vi "Get All Algorithms Info.vi"(6 "Backend engine":T1, 8 "error in":errorcluster) -> (0 "error out":errorcluster, 3 "All Algorithms Info":T2[](array[typedef]))   [LabVIEW 2013, in "QWTBLVLib.lvlib"]
doc: "Get informations on all available Algorithms."
uses:
  QWTBLVLib.lvlib
  TD Algorithm Information.ctl
  TD Algorithm Information Input.ctl
  TD Algorithm Information Output.ctl
  TD Backend Engine.ctl
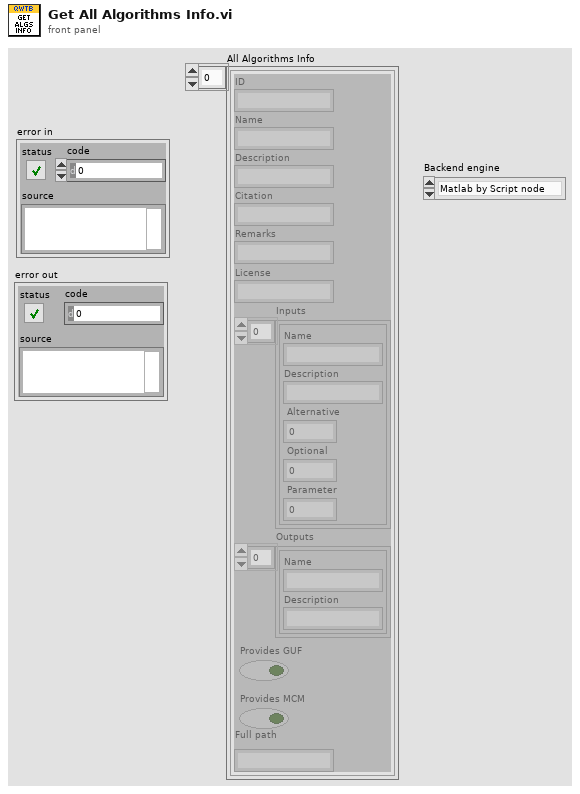
[diagram p1: front panel]
types:
  T1 = typedef "QWTBLVLib.lvlib/TD Backend Engine.ctl" = enum16{"Matlab by Script node", "GNU Octave by GOLPI"}
  T2 = typedef "QWTBLVLib.lvlib/TD Algorithm Information.ctl" = cluster{"ID":string, "Name":string, "Description":string, "Citation":string, "Remarks":string, "License":string, "Inputs":T3[], "Outputs":T4[], "Provides GUF":bool, "Provides MCM":bool, "Full path":string}
  T3 = typedef "QWTBLVLib.lvlib/TD Algorithm Information Input.ctl" = cluster{"Name":string, "Description":string, "Alternative":i32, "Optional":i32, "Parameter":i32}
  T4 = typedef "QWTBLVLib.lvlib/TD Algorithm Information Output.ctl" = cluster{"Name":string, "Description":string}
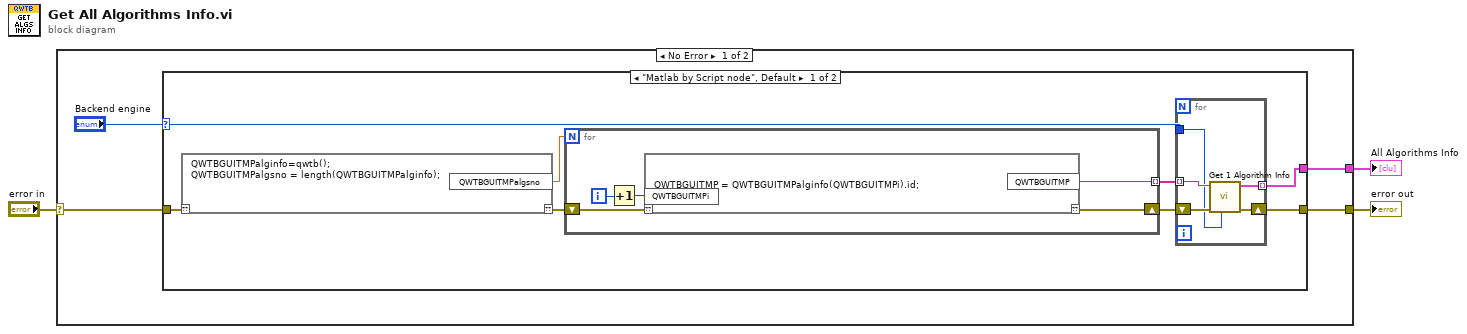
[diagram p0: block diagram]
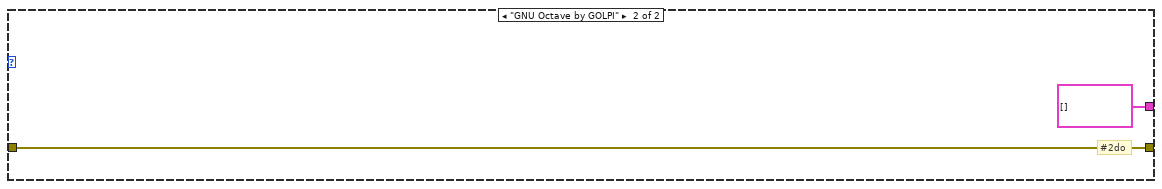
[diagram p2: hidden frame]
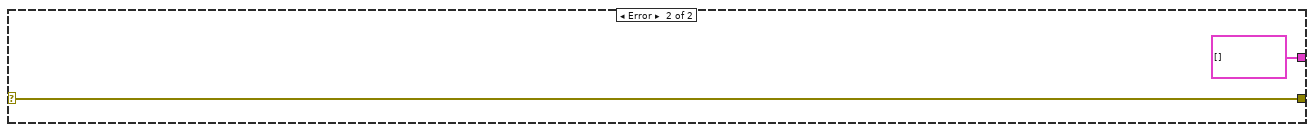
[diagram p3: hidden frame]
diagram:
  n1 = case shown="No Error" "error in" {
    selector: "error in" -> [w6 w29]
    tunnel: [w7 T2[] []] -> w3
    tunnel: [w5 w29] -> w1
    frame No Error {
      n2 = case shown="\"Matlab by Script node\", Default" "Backend engine" {
        selector: "Backend engine" -> [w8 _]
        tunnel: [w15 T2[] []] -> w7
        tunnel: w6 -> [w14 w27]
        tunnel: [w13 w27] -> w5
        frame "Matlab by Script node", Default {
          n3 = script code="QWTBGUITMPalginfo=qwtb();\nQWTBGUITMPalgsno = length(QWTBGUITMPalginfo);"("??"=w14) -> ("??"=w12:errorcluster, "QWTBGUITMPalgsno"=w9:dbl)
          n4 = for {
            N: w9 -> [_]
            tunnel: [w20] -> w10 mode=indexing
            shift-right: [w18] -> w11
            shift-left: w12 -> [w19]
            i -> [w17]
            n5 = Increment(x=w17) -> (x+1=w16:i32)
            n6 = script code="QWTBGUITMP = QWTBGUITMPalginfo(QWTBGUITMPi).id;"("??"=w19, "QWTBGUITMPi"=w16) -> ("??"=w18:errorcluster, "QWTBGUITMP"=w20:string)
          }
          n7 = for {
            tunnel: [w24] -> w15 mode=indexing
            shift-right: [w25] -> w13
            shift-left: w11 -> [w23]
            tunnel: w10 -> [w22] mode=indexing
            tunnel: w8 -> [w21]
            n8 = call "Get 1 Algorithm Info.vi"("Backend engine"=w21, "error in (no error)"=w23, "Algorithm ID"=w22) -> ("error out"=w25:errorcluster, "Algorithm Information"=w24:T2)  [unwired: 7 in]
          }
        }
        frame "GNU Octave by GOLPI" {
          # "#2do"
        }
      }
    }
    frame Error {
    }
  }
  "All Algorithms Info" <- w3
  "error out" <- w1
